vi "9219_Pt100_Raw_to_Temp.vi"(11 "Raw Data":u32) -> (3 "Temperature (ºC)":dbl)   [LabVIEW 2019]
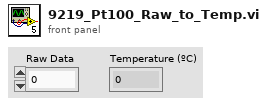
[diagram p1: front panel]
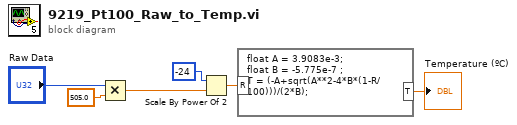
[diagram p0: block diagram]
diagram:
  n1 = Multiply(x="Raw Data", y=505.0) -> (x*y=w1:dbl)
  n2 = Scale By Power Of 2(n=i16 -24, x=w1) -> (x*2^n=w6:dbl)
  n3 = formula code="float A = 3.9083e-3;\nfloat B = -5.775e-7 ;\nT = (-A+sqrt(A**2-4*B*(1-R/100)))/(2*B);"("R"=w6) -> ("T"=→"Temperature (ºC)":dbl)
